vi "MRAWFileSaveSample.vi"() -> ()   [LabVIEW 2015]
panel:
  out "Status":string
  out "IsRecord":bool
  in  "Command":bool
  out "Picture":picture
  out "ChildNo":u32=1
  out "DeviceNo":u32
  in  "Stop":bool
  out "Error_Out":T1
  out "Color Type":enum16{"MONO", "COLOR"}(ring)
  out "Resolution":cluster{"Width":u32, "Height":u32}
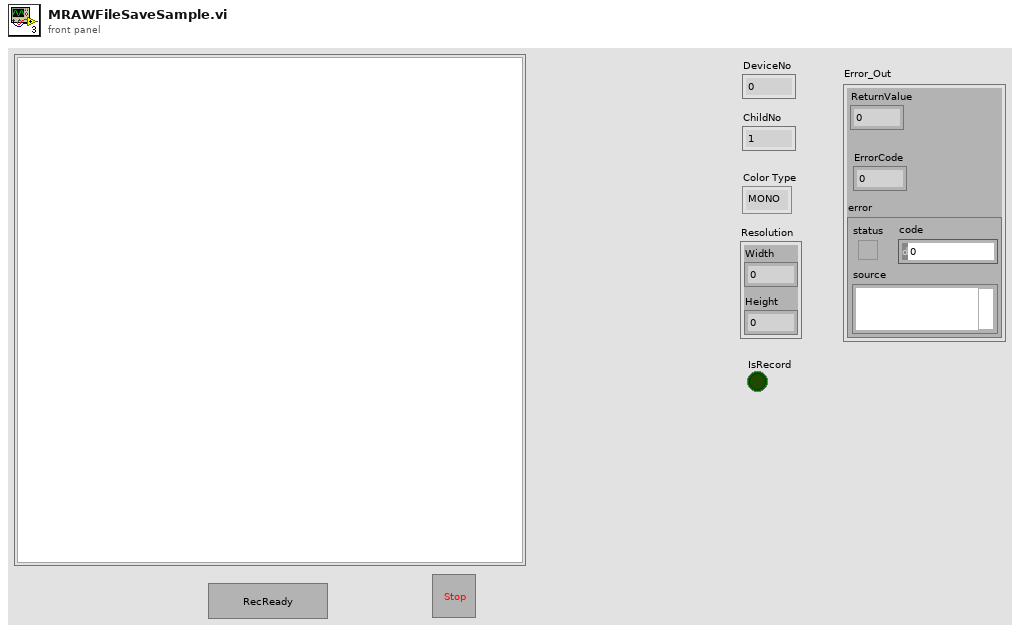
[diagram p1: front panel]
types:
  T1 = cluster{"ReturnValue":u32, "ErrorCode":u32, "error ":errorcluster}
  T2 = enum16{"Initialize", "Device Initialize", "Update Window", "Save Image", "Default", "Exit", "Error"}
  T3 = typedef "LVBoundsTypeDef.ctl" = cluster{"Width":u32, "Height":u32}
  T4 = cluster{"Start":i32, "End":i32, "Trigger":i32, "TwoStageLowToHigh":i32, "TwoStageHighToLow":i32, "TwoStageTiming":u32, "Event":i32[], "EventCount":u32, "RecordedFrames":u32}
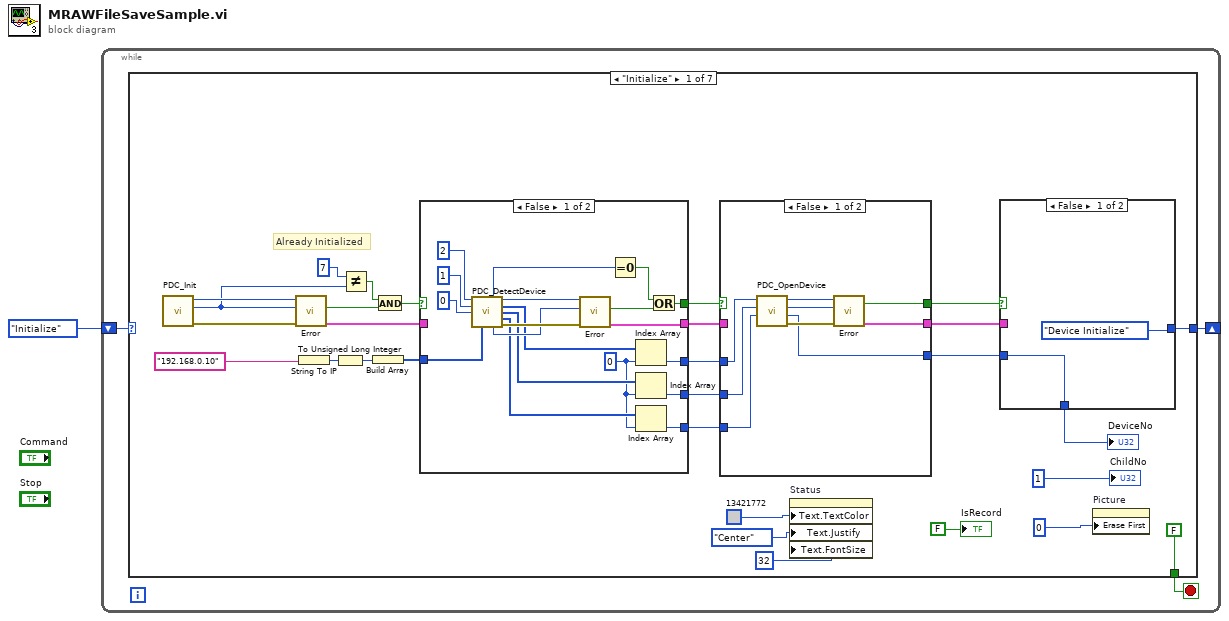
[diagram p0: block diagram]
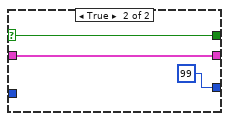
[diagram p2: hidden frame]
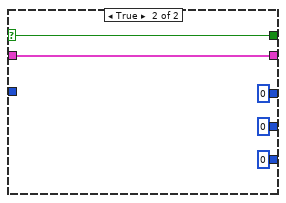
[diagram p3: hidden frame]
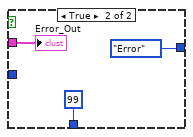
[diagram p4: hidden frame]
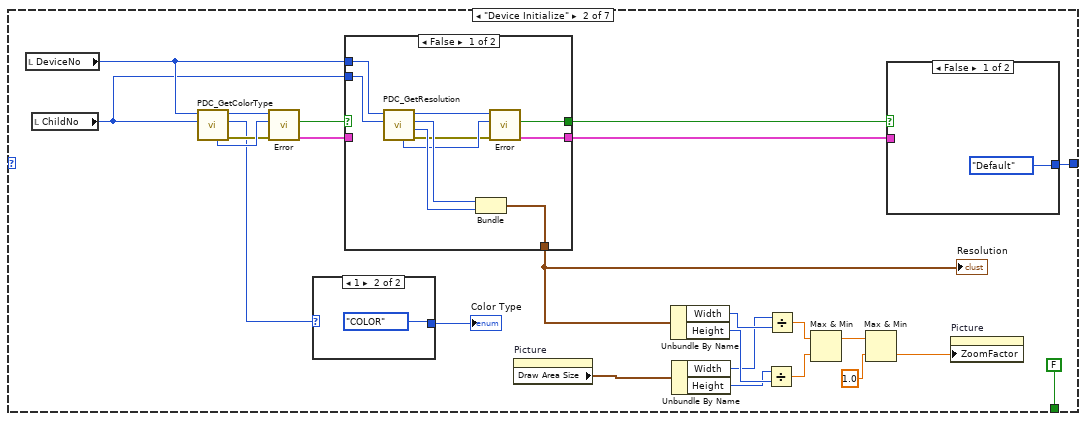
[diagram p5: hidden frame]
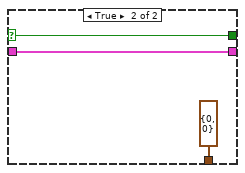
[diagram p6: hidden frame]
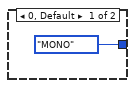
[diagram p7: hidden frame]
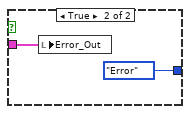
[diagram p8: hidden frame]
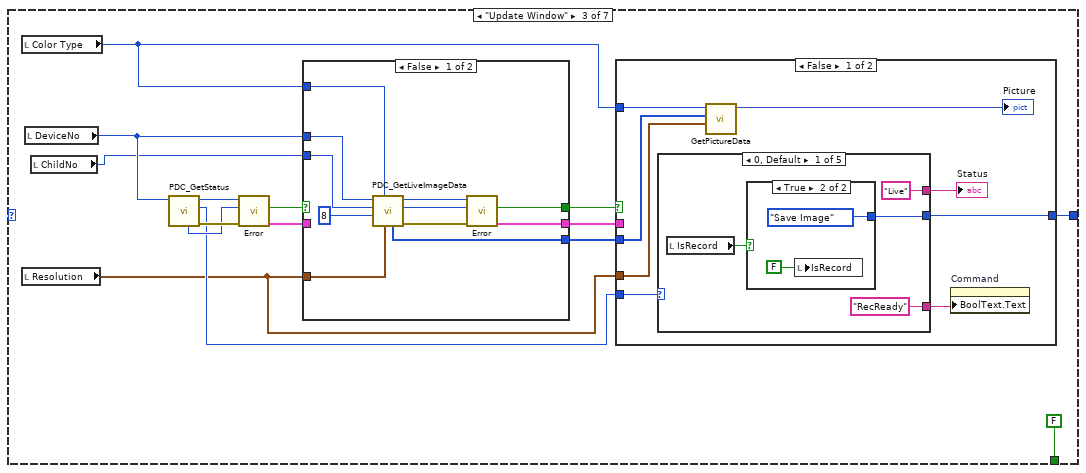
[diagram p9: hidden frame]
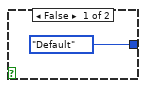
[diagram p10: hidden frame]
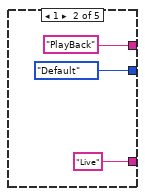
[diagram p11: hidden frame]
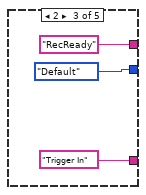
[diagram p12: hidden frame]
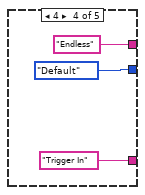
[diagram p13: hidden frame]
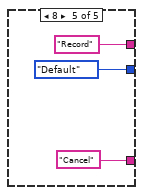
[diagram p14: hidden frame]
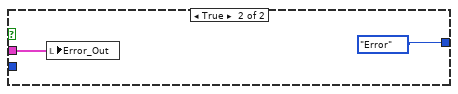
[diagram p15: hidden frame]
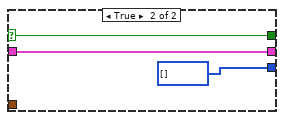
[diagram p16: hidden frame]
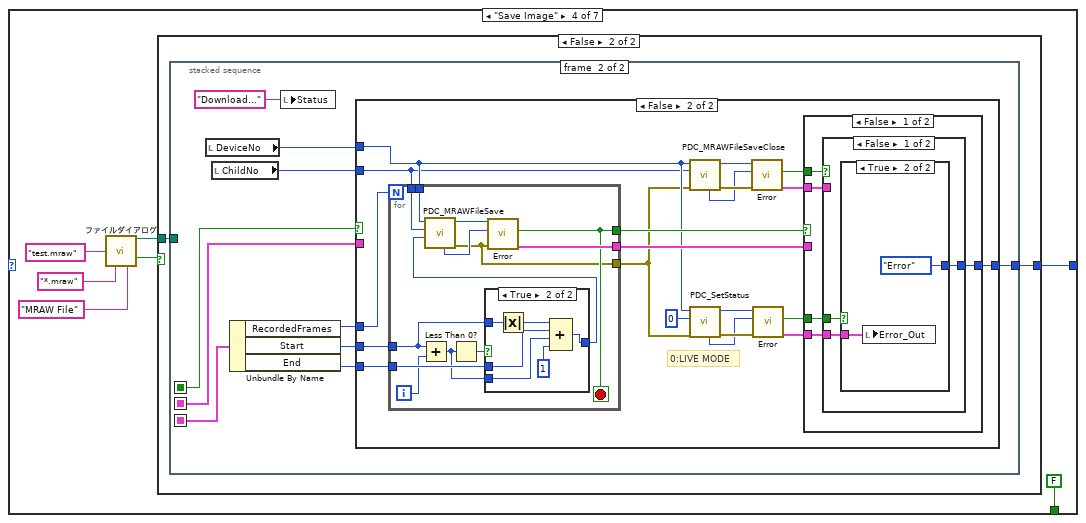
[diagram p17: hidden frame]
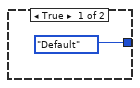
[diagram p18: hidden frame]
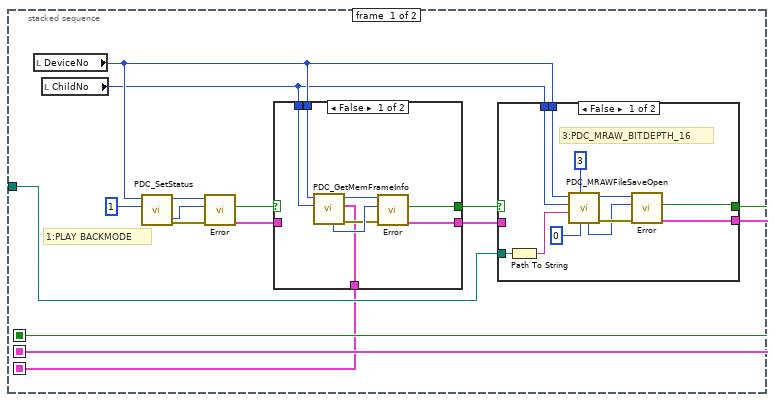
[diagram p19: hidden frame]
diagram:
  n1 = while {
    shift-right: [w2] -> _
    shift-left: T2."Initialize" ("Mode") -> [w4]
    stop <- w3 stop-if-true
    n2 = case shown="\"Initialize\"" w4 {
      tunnel: [FALSE FALSE FALSE FALSE FALSE TRUE FALSE] -> w3
      tunnel: [w12 w88 w122 w175 w289 _ T2."Exit" ("Mode")] -> w2
      frame "Initialize" {
        # "Already Initialized"
        n3 = call "PDC_Init.vi"() -> ("error out"=w33:errorcluster, "ErrorCode"=w29:u32, "ReturnValue"=w32:u32)  [unwired: 9 in]
        n4 = call "Error.vi"("error in (no error)"=w33, "ErrorCode"=w29, "ReturnValue"=w32) -> ("Error_Out"=w26:T1, "Error?"=w31:bool)  [unwired: 7 in]
        n5 = String To IP(1:"192.168.0.10") -> (0:w19:u32)
        n6 = To Unsigned Long Integer(number=w19) -> (unsigned 32bit integer=w20:u32)
        n7 = Not Equal?(x=u32 7, y=w29) -> (x != y?=w30:bool)
        n8 = Build Array(w20) -> (w17:u32[])
        n9 = And(x=w30, y=w31) -> (x .and. y?=w27:bool)
        n10 = case shown="False" w27 {
          selector: w27 -> [_ w68]
          tunnel: w26 -> [_ w69]
          tunnel: [w56 w69] -> w24
          tunnel: [w58 w68] -> w25
          tunnel: w17 -> [w53 _]
          tunnel: [w48 u32 0 ("m_nDeviceCode")] -> w16
          tunnel: [w47 u32 0 ("m_nTmpDeviceNo")] -> w15
          tunnel: [w46 u32 0] -> w14
          frame False {
            w49 = 0 ("指標")
            n11 = call "PDC_DetectDevice.vi"("InterfaceCode"=u32 2, "DetectNum"=u32 1, "DetectParam"=u32 0, "DetectNo"=w53) -> ("DeviceNum"=w54:u32, "ReturnValue"=w60:u32, "DeviceCode"=w52:u32[], "TmpDeviceNo"=w51:u32[], "InterfaceCode(out)"=w50:u32[], "ErrorCode"=w59:u32, "error out"=w61:errorcluster)  [unwired: 5 in]
            n12 = call "Error.vi"("error in (no error)"=w61, "ErrorCode"=w59, "ReturnValue"=w60) -> ("Error_Out"=w56:T1, "Error?"=w57:bool)  [unwired: 7 in]
            n13 = Equal To 0?(x=w54) -> (x = 0?=w55:bool)
            n14 = Index Array(array=w52, index=w49) -> (element=w48:u32)
            n15 = Index Array(array=w51, index=w49) -> (element=w47:u32)
            n16 = Index Array(array=w50, index=w49) -> (element=w46:u32)
            n17 = Or(x=w55, y=w57) -> (x .or. y?=w58:bool)
          }
          frame True {
          }
        }
        n18 = case shown="False" w25 {
          selector: w25 -> [_ w44]
          tunnel: w24 -> [_ w45]
          tunnel: [w42 w45] -> w21
          tunnel: [w35 w44] -> w22
          tunnel: w16 -> [w36 _]
          tunnel: w15 -> [w37 _]
          tunnel: w14 -> [w38 _]
          tunnel: [w34 u32 99 ("DeviceNo")] -> w13
          frame False {
            n19 = call "PDC_OpenDevice.vi"("InterfaceCode"=w38, "TmpDeviceNo"=w37, "DeviceCode"=w36) -> ("error out"=w41:errorcluster, "DeviceNo"=w34:u32, "ErrorCode"=w39:u32, "ReturnValue"=w40:u32)  [unwired: 5 in]
            n20 = call "Error.vi"("error in (no error)"=w41, "ErrorCode"=w39, "ReturnValue"=w40) -> ("Error_Out"=w42:T1, "Error?"=w35:bool)  [unwired: 7 in]
          }
          frame True {
          }
        }
        n21 = property on="Status" class="Str"("Text.TextColor"=u32 13421772, "Text.Justify"=enum16{"Left", "Center", "Right"}."Center" ("テキスト.位置調整"), "Text.FontSize"=u32 32 ("テキスト.フォント:サイズ")) -> ()  [unwired: 2 in, 2 out]
        n22 = case shown="False" w22 {
          tunnel: [T2."Device Initialize" ("Mode") T2."Error" ("Mode")] -> w12
          tunnel: w21 -> [_ w72]
          tunnel: w13 -> [w71 _]
          tunnel: [w71 u32 99 ("DeviceNo")] -> w9
          frame False {
          }
          frame True {
            "Error_Out" <- w72
          }
        }
        "DeviceNo" <- w9
        n23 = property on="Picture" class="Pict"("Erase First"=u8 0 ("最初に削除")) -> ()  [unwired: 2 in, 2 out]
        "IsRecord" <- FALSE ("IsRecord")
        "ChildNo" <- u32 1
      }
      frame "Device Initialize" {
        n24 = local read "DeviceNo"() -> (w87:u32)
        n25 = local read "ChildNo"() -> (w86:u32)
        n26 = call "PDC_GetColorType.vi"("ChildNo"=w86, "DeviceNo"=w87) -> ("error out"=w96:errorcluster, "Mode"=w95:i8, "ReturnValue"=w98:u32, "ErrorCode"=w97:u32)  [unwired: 6 in]
        n27 = call "Error.vi"("error in (no error)"=w96, "ErrorCode"=w97, "ReturnValue"=w98) -> ("Error_Out"=w92:T1, "Error?"=w93:bool)  [unwired: 7 in]
        n28 = case shown="1" w95 {
          tunnel: [enum16{"MONO", "COLOR"}."MONO" enum16{"MONO", "COLOR"}."COLOR"] -> w94
          frame 0, Default {
          }
          frame 1 {
          }
        }
        "Color Type" <- w94
        n29 = case shown="False" w93 {
          selector: w93 -> [_ w110]
          tunnel: w92 -> [_ w111]
          tunnel: [w102 w111] -> w89
          tunnel: [w103 w110] -> w90
          tunnel: w87 -> [w101 _]
          tunnel: w86 -> [w100 _]
          tunnel: [w99 cluster{"Width":u32, "Height":u32} {"Width"=0, "Height"=0}] -> w77
          frame False {
            n30 = call "PDC_GetResolution.vi"("ChildNo"=w100, "DeviceNo"=w101) -> ("error out"=w105:errorcluster, "Height"=w108:u32, "Width"=w107:u32, "ReturnValue"=w104:u32, "ErrorCode"=w106:u32)  [unwired: 5 in]
            n31 = Bundle("Width"=w107, "Height"=w108) -> (w99:cluster{"Width":u32, "Height":u32})  [unwired: 1 in]
            n32 = call "Error.vi"("error in (no error)"=w105, "ErrorCode"=w106, "ReturnValue"=w104) -> ("Error_Out"=w102:T1, "Error?"=w103:bool)  [unwired: 7 in]
          }
          frame True {
          }
        }
        "Resolution" <- w77
        n33 = property on="Picture" class="Pict"() -> ("Draw Area Size"=w76:T3)  [unwired: 2 in, 2 out]
        n34 = Unbundle By Name(w77) -> ("Width"=w85:u32, "Height"=w84:u32)
        n35 = Unbundle By Name(w76) -> ("Width"=w83:u32, "Height"=w82:u32)
        n36 = Divide(x=w82, y=w84) -> (x/y=w80:dbl)
        n37 = Divide(x=w83, y=w85) -> (x/y=w81:dbl)
        n38 = Max & Min(x=w81, y=w80) -> (max(x,y)=w79:dbl)  [unwired: 1 out]
        n39 = Max & Min(x=w79, y=1.0) -> (min(x,y)=w75:dbl)  [unwired: 1 out]
        n40 = case shown="False" w90 {
          tunnel: [T2."Default" ("Mode") T2."Error" ("Mode")] -> w88
          tunnel: w89 -> [_ w115]
          frame False {
          }
          frame True {
            n41 = local write "Error_Out"(w115) -> ()
          }
        }
        n42 = property on="Picture" class="Pict"("ZoomFactor"=w75) -> ()  [unwired: 2 in, 2 out]
      }
      frame "Update Window" {
        n43 = local read "Color Type"() -> (w120:enum16{"MONO", "COLOR"})
        n44 = local read "Resolution"() -> (w117:cluster{"Width":u32, "Height":u32})
        n45 = local read "DeviceNo"() -> (w119:u32)
        n46 = local read "ChildNo"() -> (w118:u32)
        n47 = call "PDC_GetStatus.vi"("DeviceNo"=w119) -> ("error out"=w131:errorcluster, "Status"=w121:u32, "ReturnValue"=w130:u32, "ErrorCode"=w128:u32)  [unwired: 7 in]
        n48 = call "Error.vi"("error in (no error)"=w131, "ErrorCode"=w128, "ReturnValue"=w130) -> ("Error_Out"=w127:T1, "Error?"=w129:bool)  [unwired: 7 in]
        n49 = case shown="False" w129 {
          selector: w129 -> [_ w173]
          tunnel: w127 -> [_ w174]
          tunnel: [w171 w174] -> w125
          tunnel: [w169 w173] -> w124
          tunnel: w119 -> [w166 _]
          tunnel: w118 -> [w165 _]
          tunnel: [w163 u8[] [] ("Data(8Bit)")] -> w123
          tunnel: w120 -> [w162 _]
          tunnel: w117 -> [w161 _]
          frame False {
            n50 = call "PDC_GetLiveImageData.vi"("Resolution"=w161, "ColorType"=w162, "BitDepth"=u32 8, "ChildNo"=w165, "DeviceNo"=w166) -> ("error out"=w170:errorcluster, "ErrorCode"=w167:u32, "ReturnValue"=w168:u32, "Data(8Bit)"=w163:u8[])  [unwired: 2 in, 1 out]
            n51 = call "Error.vi"("error in (no error)"=w170, "ErrorCode"=w167, "ReturnValue"=w168) -> ("Error_Out"=w171:T1, "Error?"=w169:bool)  [unwired: 7 in]
          }
          frame True {
          }
        }
        n52 = case shown="False" w124 {
          tunnel: w125 -> [_ w159]
          tunnel: w123 -> [w138 _]
          tunnel: w121 -> [w136 _]
          tunnel: [w134 T2."Error" ("Mode")] -> w122
          tunnel: w117 -> [w137 _]
          tunnel: w120 -> [w139 _]
          frame False {
            n53 = case shown="0, Default" w136 {
              tunnel: ["Live" "PlayBack" "RecReady" "Endless" "Record"] -> w132
              tunnel: ["RecReady" "Live" "Trigger In" "Trigger In" "Cancel"] -> w135
              tunnel: [w141 T2."Default" ("Mode") T2."Default" ("Mode") T2."Default" ("Mode") T2."Default" ("Mode")] -> w134
              frame 0, Default {
                n54 = local read "IsRecord"() -> (w140:bool)
                n55 = case shown="True" w140 {
                  tunnel: [T2."Default" ("Mode") T2."Save Image" ("Mode")] -> w141
                  frame False {
                  }
                  frame True {
                    n56 = local write "IsRecord"(FALSE ("IsRecord")) -> ()
                  }
                }
              }
              frame 1 {
              }
              frame 2 {
              }
              frame 4 {
              }
              frame 8 {
              }
            }
            "Status" <- w132
            n57 = call "GetPictureData.vi"("Resolution"=w137, "Data(8Bit)"=w138, "ColorType"=w139) -> ("new picture"=→"Picture":picture)  [unwired: 4 in]
            n58 = property on="Command" class="Bool (strict)"("BoolText.Text"=w135) -> ()  [unwired: 2 in, 2 out]
          }
          frame True {
            n59 = local write "Error_Out"(w159) -> ()
          }
        }
      }
      frame "Save Image" {
        n60 = call "ファイルダイアログ"("default name"="test.mraw", "pattern (all files)"="*.mraw", "pattern label"="MRAW File") -> ("selected path"=w176:path, "cancelled"=w177:bool)  [unwired: 9 in, 2 out]
        n61 = case shown="False" w177 {
          tunnel: w176 -> [_ w184]
          tunnel: [T2."Default" ("Mode") w183] -> w175
          frame True {
          }
          frame False {
            n62 = stacked-sequence {
              seq-local: [w189 _] -> [_ w228]
              seq-local: [w188 _] -> [_ w227]
              seq-local: [w187 _] -> [_ w223]
              tunnel: w184 -> [w190 _]
              tunnel: [_ w231] -> w183
              frame #0 {
                # "1:PLAY BACKMODE"
                n63 = local read "DeviceNo"() -> (w186:u32)
                n64 = local read "ChildNo"() -> (w185:u32)
                n65 = call "PDC_SetStatus.vi"("Mode"=u32 1, "DeviceNo"=w186) -> ("error out"=w197:errorcluster, "ReturnValue"=w198:u32, "ErrorCode"=w196:u32)  [unwired: 7 in]
                n66 = call "Error.vi"("error in (no error)"=w197, "ErrorCode"=w196, "ReturnValue"=w198) -> ("Error_Out"=w193:T1, "Error?"=w194:bool)  [unwired: 7 in]
                n67 = case shown="False" w194 {
                  selector: w194 -> [_ w221]
                  tunnel: [w216 w220] -> w191
                  tunnel: [w215 w221] -> w192
                  tunnel: [w214 _] -> w187
                  tunnel: w193 -> [_ w220]
                  tunnel: w186 -> [w213 _]
                  tunnel: w185 -> [w212 _]
                  frame False {
                    n68 = call "PDC_GetMemFrameInfo.vi"("ChildNo"=w212, "DeviceNo"=w213) -> ("error out"=w217:errorcluster, "Frame"=w214:T4, "ReturnValue"=w218:u32, "ErrorCode"=w219:u32)  [unwired: 6 in]
                    n69 = call "Error.vi"("error in (no error)"=w217, "ErrorCode"=w219, "ReturnValue"=w218) -> ("Error_Out"=w216:T1, "Error?"=w215:bool)  [unwired: 7 in]
                  }
                  frame True {
                  }
                }
                n70 = case shown="False" w192 {
                  selector: w192 -> [_ w211]
                  tunnel: w191 -> [_ w210]
                  tunnel: [w203 w211] -> w189
                  tunnel: [w204 w210] -> w188
                  tunnel: w190 -> [w202 _]
                  tunnel: w186 -> [w200 _]
                  tunnel: w185 -> [w199 _]
                  frame False {
                    # "3:PDC_MRAW_BITDEPTH_16"
                    n71 = Path To String(path=w202) -> (string=w209:string)
                    n72 = call "PDC_MRAWFileSaveOpen.vi"("MaxFrameNum"=0, "MRawBitDepth"=u32 3, "FileName"=w209, "ChildNo"=w199, "DeviceNo"=w200) -> ("error out"=w208:errorcluster, "ReturnValue"=w207:u32, "ErrorCode"=w206:u32)  [unwired: 4 in]
                    n73 = call "Error.vi"("error in (no error)"=w208, "ErrorCode"=w206, "ReturnValue"=w207) -> ("Error_Out"=w204:T1, "Error?"=w203:bool)  [unwired: 7 in]
                  }
                  frame True {
                  }
                }
              }
              frame #1 {
                n74 = local read "DeviceNo"() -> (w230:u32)
                n75 = local read "ChildNo"() -> (w229:u32)
                n76 = Unbundle By Name(w223) -> ("RecordedFrames"=w226:u32, "Start"=w225:i32, "End"=w224:i32)
                n77 = local write "Status"("Download..." ("Status")) -> ()
                n78 = case shown="False" w228 {
                  tunnel: w227 -> [w232 _]
                  tunnel: w230 -> [_ w236]
                  tunnel: w229 -> [_ w235]
                  tunnel: w226 -> [_ w253]
                  tunnel: w225 -> [_ w252]
                  tunnel: w224 -> [_ w251]
                  tunnel: [T2."Error" ("Mode") w237] -> w231
                  frame True {
                    n79 = local write "Error_Out"(w232) -> ()
                  }
                  frame False {
                    # "0:LIVE MODE"
                    n80 = for "Forループ" {
                      N: w253 -> [_]
                      tunnel: w252 -> [w272]
                      tunnel: w251 -> [w277]
                      tunnel: [w275] -> w243
                      tunnel: [w276] -> w242
                      tunnel: w236 -> [w274]
                      tunnel: w235 -> [w273]
                      tunnel: [w269] -> w234
                      i -> [w271]
                      stop <- w275 stop-if-true
                      n81 = Add(x=w272, y=w271) -> (x+y=w270:i32)
                      n82 = Less Than 0?(x=w270) -> (x < 0?=w279:bool)
                      n83 = case shown="True" w279 {
                        tunnel: w270 -> [w282 w285]
                        tunnel: [w282 w283] -> w278
                        tunnel: w277 -> [_ w286]
                        tunnel: w272 -> [_ w288]
                        frame False {
                        }
                        frame True {
                          n84 = Absolute Value(x=w288) -> (abs(x)=w287:i32)
                          n85 = Compound Arithmetic op=ADD(w287, w286, w285, 1 ("値")) -> (w283:i32)
                        }
                      }
                      n86 = call "PDC_MRAWFileSave.vi"("FrameNo"=w278, "ChildNo"=w273, "DeviceNo"=w274) -> ("error out"=w269:errorcluster, "ReturnValue"=w281:u32, "ErrorCode"=w280:u32)  [unwired: 6 in]
                      n87 = call "Error.vi"("error in (no error)"=w269, "ErrorCode"=w280, "ReturnValue"=w281) -> ("Error_Out"=w276:T1, "Error?"=w275:bool)  [unwired: 7 in]
                    }
                    n88 = call "PDC_MRAWFileSaveClose.vi"("error in (no error)"=w234, "ChildNo"=w235, "DeviceNo"=w236) -> ("error out"=w249:errorcluster, "ReturnValue"=w250:u32, "ErrorCode"=w248:u32)  [unwired: 6 in]
                    n89 = call "PDC_SetStatus.vi"("error in (no error)"=w234, "Mode"=u32 0 ("ChildNo"), "DeviceNo"=w236) -> ("error out"=w246:errorcluster, "ReturnValue"=w247:u32, "ErrorCode"=w245:u32)  [unwired: 6 in]
                    n90 = call "Error.vi"("error in (no error)"=w249, "ErrorCode"=w248, "ReturnValue"=w250) -> ("Error_Out"=w240:T1, "Error?"=w241:bool)  [unwired: 7 in]
                    n91 = call "Error.vi"("error in (no error)"=w246, "ErrorCode"=w245, "ReturnValue"=w247) -> ("Error_Out"=w238:T1, "Error?"=w239:bool)  [unwired: 7 in]
                    n92 = case shown="False" w243 {
                      tunnel: w242 -> [_ w267]
                      tunnel: [w256 T2."Error" ("Mode")] -> w237
                      tunnel: w241 -> [w258 _]
                      tunnel: w240 -> [w257 _]
                      tunnel: w239 -> [w255 _]
                      tunnel: w238 -> [w254 _]
                      frame False {
                        n93 = case shown="False" w258 {
                          tunnel: w257 -> [_ w265]
                          tunnel: [w259 T2."Error" ("Mode")] -> w256
                          tunnel: w255 -> [w261 _]
                          tunnel: w254 -> [w260 _]
                          frame False {
                            n94 = case shown="True" w261 {
                              tunnel: w260 -> [_ w263]
                              tunnel: [T2."Default" ("Mode") T2."Error" ("Mode")] -> w259
                              frame False {
                              }
                              frame True {
                                n95 = local write "Error_Out"(w263) -> ()
                              }
                            }
                          }
                          frame True {
                            n96 = local write "Error_Out"(w265) -> ()
                          }
                        }
                      }
                      frame True {
                        n97 = local write "Error_Out"(w267) -> ()
                      }
                    }
                  }
                }
              }
            }
          }
        }
      }
      frame "Default" {
        n98 = event shown="[1] \"Command\": Value Change" {
          selector: _ -> [_ _ _]
          dyn-events: _ -> [_ _ _]
          timeout: 10 -> [_ _ _]
          tunnel: [T2."Update Window" ("Mode") w293 T2."Exit" ("Mode")] -> w289
          event Timeout {
            n99 = event-data() -> ()  [unwired: 1 in, 2 out]
          }
          event "Command": Value Change {
            n100 = event-data() -> ("NewVal"=w294:bool)  [unwired: 1 in, 4 out]
            n101 = case shown="True" w294 {
              tunnel: [T2."Default" ("Mode") w297] -> w293
              frame False {
              }
              frame True {
                n102 = local read "DeviceNo"() -> (w296:u32)
                n103 = call "PDC_GetStatus.vi"("DeviceNo"=w296) -> ("error out"=w305:errorcluster, "Status"=w300:u32, "ReturnValue"=w304:u32, "ErrorCode"=w303:u32)  [unwired: 7 in]
                n104 = call "Error.vi"("error in (no error)"=w305, "ErrorCode"=w303, "ReturnValue"=w304) -> ("Error_Out"=w301:T1, "Error?"=w302:bool)  [unwired: 7 in]
                n105 = case shown="False" w302 {
                  selector: w302 -> [_ w347]
                  tunnel: w301 -> [_ w348]
                  tunnel: [w310 w348] -> w298
                  tunnel: [w309 w347] -> w299
                  tunnel: w300 -> [w312 _]
                  tunnel: w296 -> [w311 _]
                  frame False {
                    n106 = case shown="0, Default" w312 {
                      tunnel: w311 -> [w313 w321 w327 w334 w342]
                      tunnel: [w318 w325 w332 w339 w346] -> w310
                      tunnel: [w317 w324 w331 w338 w345] -> w309
                      frame 0, Default {
                        n107 = call "PDC_SetRecReady.vi"("DeviceNo"=w313) -> ("error out"=w316:errorcluster, "ReturnValue"=w315:u32, "ErrorCode"=w314:u32)  [unwired: 8 in]
                        n108 = call "Error.vi"("error in (no error)"=w316, "ErrorCode"=w314, "ReturnValue"=w315) -> ("Error_Out"=w318:T1, "Error?"=w317:bool)  [unwired: 7 in]
                      }
                      frame 1 {
                        n109 = call "PDC_SetStatus.vi"("Mode"=u32 0, "DeviceNo"=w321) -> ("error out"=w323:errorcluster, "ReturnValue"=w322:u32, "ErrorCode"=w320:u32)  [unwired: 7 in]
                        n110 = call "Error.vi"("error in (no error)"=w323, "ErrorCode"=w320, "ReturnValue"=w322) -> ("Error_Out"=w325:T1, "Error?"=w324:bool)  [unwired: 7 in]
                      }
                      frame 2 {
                        n111 = call "PDC_TriggerIn.vi"("DeviceNo"=w327) -> ("error out"=w330:errorcluster, "ReturnValue"=w329:u32, "ErrorCode"=w328:u32)  [unwired: 8 in]
                        n112 = call "Error.vi"("error in (no error)"=w330, "ErrorCode"=w328, "ReturnValue"=w329) -> ("Error_Out"=w332:T1, "Error?"=w331:bool)  [unwired: 7 in]
                        n113 = local write "IsRecord"(TRUE ("IsRecord")) -> ()
                      }
                      frame 4 {
                        n114 = call "PDC_TriggerIn.vi"("DeviceNo"=w334) -> ("error out"=w337:errorcluster, "ReturnValue"=w336:u32, "ErrorCode"=w335:u32)  [unwired: 8 in]
                        n115 = call "Error.vi"("error in (no error)"=w337, "ErrorCode"=w335, "ReturnValue"=w336) -> ("Error_Out"=w339:T1, "Error?"=w338:bool)  [unwired: 7 in]
                        n116 = local write "IsRecord"(TRUE ("IsRecord")) -> ()
                      }
                      frame 8 {
                        n117 = call "PDC_SetStatus.vi"("Mode"=u32 0, "DeviceNo"=w342) -> ("error out"=w344:errorcluster, "ReturnValue"=w343:u32, "ErrorCode"=w341:u32)  [unwired: 7 in]
                        n118 = call "Error.vi"("error in (no error)"=w344, "ErrorCode"=w341, "ReturnValue"=w343) -> ("Error_Out"=w346:T1, "Error?"=w345:bool)  [unwired: 7 in]
                      }
                    }
                  }
                  frame True {
                  }
                }
                n119 = case shown="False" w299 {
                  tunnel: w298 -> [_ w307]
                  tunnel: [T2."Default" ("Mode") T2."Error" ("Mode")] -> w297
                  frame False {
                  }
                  frame True {
                    n120 = local write "Error_Out"(w307) -> ()
                  }
                }
              }
            }
          }
          event "Stop": Value Change {
            n121 = event-data() -> ()  [unwired: 1 in, 5 out]
          }
        }
      }
      frame "Exit" {
        n122 = local read "DeviceNo"() -> (w350:u32)
        n123 = case shown="Default" w350 {
          selector: w350 -> [_ w352]
          frame 99 {
          }
          frame Default {
            n124 = call "PDC_CloseDevice.vi"("DeviceNo"=w352) -> ()  [unwired: 8 in, 3 out]
          }
        }
      }
      frame "Error" {
        w356 = "\r\n"
        n125 = local read "Error_Out"() -> (w353:T1)
        n126 = Unbundle By Name(w353) -> ("error"=w371:errorcluster, "error.source"=w368:string, "error.code"=w367:i32, "ReturnValue"=w364:u32, "ErrorCode"=w363:u32)
        n127 = Number To Decimal String(number=w367) -> (decimal integer string=w365:string)  [unwired: 1 out]
        n128 = Number To Decimal String(number=w364) -> (decimal integer string=w361:string)  [unwired: 1 out]
        n129 = Number To Decimal String(number=w363) -> (decimal integer string=w359:string)  [unwired: 1 out]
        n130 = call <vilib>:"Clear Errors.vi"("error in (no error)"=w371) -> ("error out"=w370:errorcluster)  [unwired: 1 in, 5 out]
        n131 = Concatenate Strings("<<Error !!>>", w356, w356, w356, "Source=", w368, w356, "LabError=", w365, w356, "ReturnType=", w361, w356, "ErrorCode=", w359) -> (w358:string)
        n132 = call "メッセージ表示"("error in (no error)"=w370, "Message"=w358) -> ()  [unwired: 1 in, 9 out]
      }
    }
  }
